vi "SetVoltageEx.vi"() -> ()   [LabVIEW 2019]
uses:
  <vilib>/Instr/_visa.llb/VISA Configure Serial Port (Instr).vi
panel:
  in  "Slide":dbl(slide) scale=0.0..16.0
  out "read buffer":string
  out "return count":u32
  in  "VISA resource name":refnum<visa-resource-name>
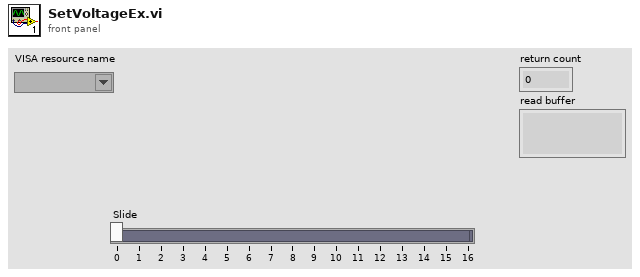
[diagram p1: front panel]
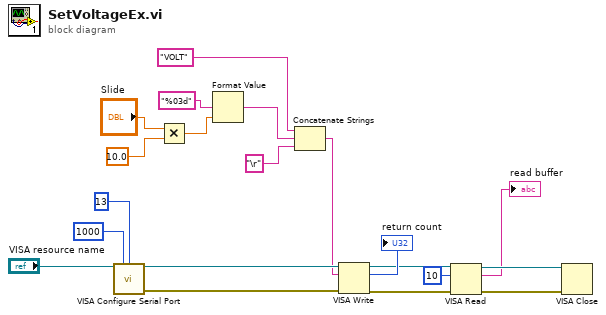
[diagram p0: block diagram]
diagram:
  n1 = call-poly "VISA Configure Serial Port"("VISA resource name"="VISA resource name", "timeout (10sec)"=u32 1000, "termination char\n(0xA = '\\n' = LF)"=u8 13 ("termination char\n(0xA = '\\n' = LF)")) -> ("VISA resource name out"=w17:refnum<visa-resource-name>, "error out"=w16:errorcluster)  [unwired: 11 in]
  n2 = Multiply(x="Slide", y=10.0) -> (x*y=w7:dbl)
  n3 = Format Value(format string="%03d", value (0)=w7) -> (output string=w3:string)  [unwired: 1 in]
  n4 = Concatenate Strings("VOLT" ("write buffer"), w3, "\r" ("string")) -> (w1:string)
  n5 = VISA Write(VISA resource name=w17, write buffer=w1, error in (no error)=w16) -> (VISA resource name out=w14:refnum<visa-resource-name>, return count=→"return count":u32, error out=w13:errorcluster)
  n6 = VISA Read(VISA resource name=w14, byte count=u32 10, error in (no error)=w13) -> (VISA resource name out=w12:refnum<visa-resource-name>, read buffer=→"read buffer":string, error out=w11:errorcluster)  [unwired: 1 out]
  n7 = VISA Close(VISA resource name=w12, error in (no error)=w11) -> ()  [unwired: 1 out]
